vi "turnOnOrOffMatchingChannels.vi"(7 "override\"Always\"chs":bool=TRUE, 9 "setState":T1, 10 "regular expression":string="VAC-1-b:") -> (1 "numMatches":i32, 2 "MatchedChannels":string[](array[string]), 3 "Channels":string[](array[string]))   [LabVIEW 2021]
uses:
  Sub VIs/ADAM Controls/Channel_names.ctl
  Sub VIs/ADAM Controls/Channel_State.ctl
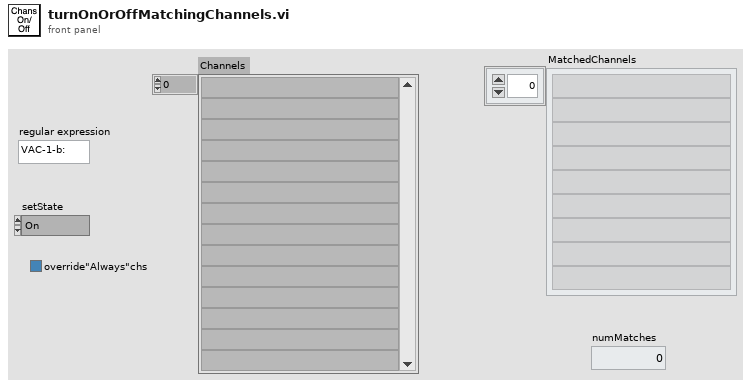
[diagram p1: front panel]
types:
  T1 = typedef "Channel_State.ctl" = enum16{"On", "Off", "Always On", "Always Off"}
  T2 = typedef "Channel_names.ctl" = enum16{"Active Only", "Active + Off", "All Channels", "Changeable Only"}
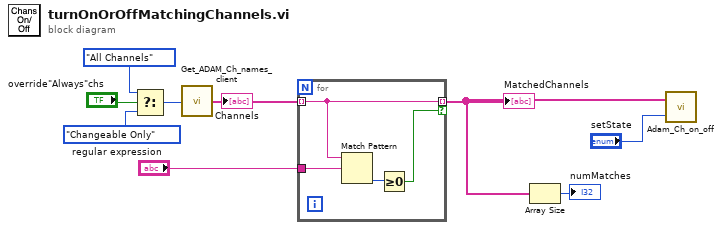
[diagram p0: block diagram]
diagram:
  n1 = Select(t=Channel_names."All Channels" ("Channel names set"), s="override\"Always\"chs", f=Channel_names."Changeable Only" ("Channel names set")) -> (s? t:f=w2:T2)
  n2 = call "Get_ADAM_Ch_names_client.vi"("Channel names set"=w2) -> ("Ch names"=w5:string[])
  "Channels" <- w5
  n3 = for {
    tunnel: [w10] -> w9 mode=indexing if=w11
    tunnel: "regular expression" -> [w12]
    tunnel: w5 -> [w10] mode=indexing
    n4 = Match Pattern(string=w10, regular expression=w12) -> (offset past match=w13:i32)  [unwired: 1 in, 3 out]
    n5 = Greater Or Equal To 0?(x=w13) -> (x >= 0?=w11:bool)
  }
  "MatchedChannels" <- w9
  n6 = Array Size(array=w9) -> (size(s)=→"numMatches":i32)
  n7 = call "Adam_Ch_on_off.vi"("Ch State"="setState", "ADAM Ch Names"=w9) -> ()  [unwired: 1 out]
